vi "Delete LogFile if Exists.vi"(7 "Log File Path":path, 8 "error in (no error)":errorcluster, 11 "Target Information":T1) -> (0 "error out":errorcluster)   [LabVIEW 2026, in "Telemetry System Tests.lvclass"]
uses:
  Telemetry System Tests.lvclass
  <vilib>/WebDAVClient/NI_WebDAV.lvlib
  <vilib>/NI/VeriStand Custom Device Testing Tools/VeriStandTestUtilities/ChassisInformation.ctl
  <vilib>/NI/VeriStand Custom Device Testing Tools/VeriStandTestUtilities/VeriStandTestUtilities.lvlib
  <vilib>/NI/VeriStand Custom Device Testing Tools/VeriStandTestUtilities/TargetInformation.ctl
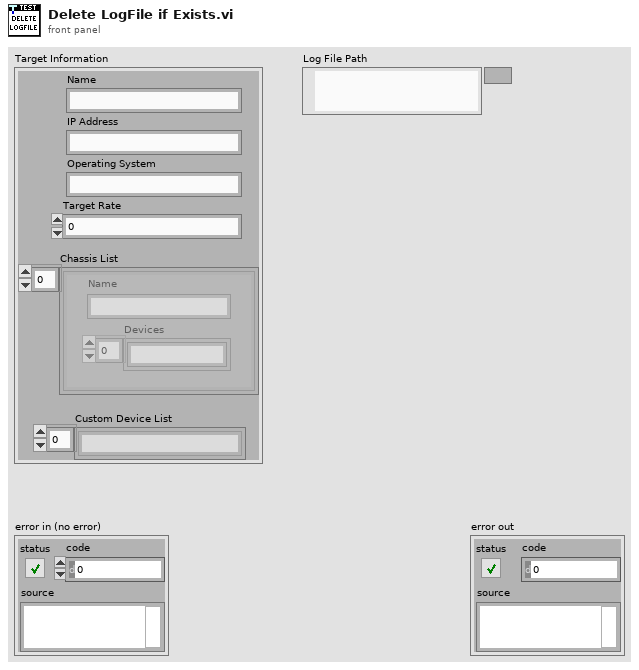
[diagram p1: front panel]
types:
  T1 = typedef "VeriStandTestUtilities.lvlib/TargetInformation.ctl" = cluster{"Name":string, "IP Address":string, "Operating System":string, "Target Rate":dbl, "Chassis List":T2[], "Custom Device List":string[]}
  T2 = typedef "VeriStandTestUtilities.lvlib/ChassisInformation.ctl" = cluster{"Name":string, "Devices":string[]}
  T3 = typedef "NI_WebDAV.lvlib/SessionHandle.ctl" = refnum<k1>
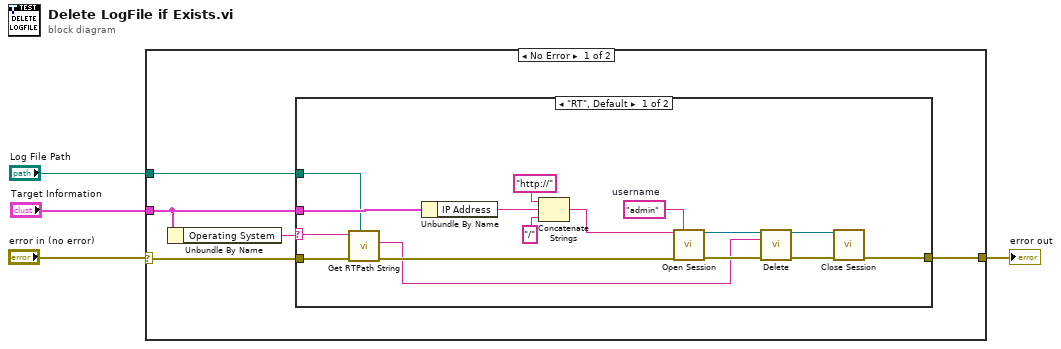
[diagram p0: block diagram]
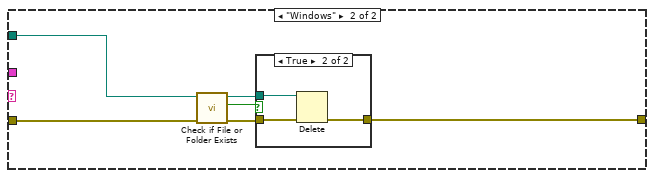
[diagram p2: hidden frame]
diagram:
  n1 = case shown="No Error" "error in (no error)" {
    selector: "error in (no error)" -> [w7 w36]
    tunnel: "Log File Path" -> [w9 _]
    tunnel: [w8 w36] -> w3
    tunnel: "Target Information" -> [w6 _]
    frame No Error {
      n2 = Unbundle By Name(w6) -> ("Operating System"=w5:string)
      n3 = case shown="\"RT\", Default" w5 {
        selector: w5 -> [w25 _]
        tunnel: [w19 w26] -> w8
        tunnel: w7 -> [w24 w30]
        tunnel: w9 -> [w11 w31]
        tunnel: w6 -> [w13 _]
        frame "RT", Default {
          w10 = "admin"  # username
          n4 = call "Get RTPath String.vi"("SysDef Log File Path"=w11, "error in (no error)"=w24, "Target OS in"=w25) -> ("error out"=w23:errorcluster, "RT File Path"=w14:string)  [unwired: 5 in, 2 out]
          n5 = Unbundle By Name(w13) -> ("IP Address"=w12:string)
          n6 = Concatenate Strings("http://" ("string"), w12, "/" ("string")) -> (w20:string)
          n7 = call <vilib>:"Open Session.vi"("host uri prefix"=w20, "username"=w10, "error in (no error)"=w23) -> ("session handle out"=w16:T3, "error out"=w18:errorcluster)  [unwired: 11 in]
          n8 = call <vilib>:"Delete.vi"("session handle"=w16, "relative uri"=w14, "error in (no error)"=w18) -> ("session handle out"=w15:T3, "error out"=w17:errorcluster)  [unwired: 11 in]
          n9 = call <vilib>:"Close Session.vi"("session handle"=w15, "error in (no error)"=w17) -> ("error out"=w19:errorcluster)  [unwired: 13 in]
        }
        frame "Windows" {
          n10 = call <vilib>:"Check if File or Folder Exists.vi"("error in (no error)"=w30, "path"=w31) -> ("error out"=w27:errorcluster, "file or folder exists?"=w28:bool, "dup path"=w29:path)  [unwired: 7 in]
          n11 = case shown="True" w28 {
            tunnel: w29 -> [_ w35]
            tunnel: w27 -> [w32 w34]
            tunnel: [w32 w33] -> w26
            frame False {
            }
            frame True {
              n12 = Delete(path (use dialog)=w35, error in=w34) -> (error out=w33:errorcluster)  [unwired: 3 in, 2 out]
            }
          }
        }
      }
    }
    frame Error {
    }
  }
  "error out" <- w3
